vi "status.vi"(8 "error in (no error)":errorcluster, 11 "EventDaemon in":refnum<class "MemoryManager.lvclass">) -> (0 "error out":errorcluster, 2 "status":T1, 3 "EventDaemon out":refnum<class "MemoryManager.lvclass">)   [LabVIEW 2024, in "MemoryManager.lvclass"]
doc: "Get current status and send via notifier."
uses:
  MemoryManager.lvclass
  status--cluster.ctl
  states--enum.ctl
  MemoryManager.lvclass/MemoryManager.ctl
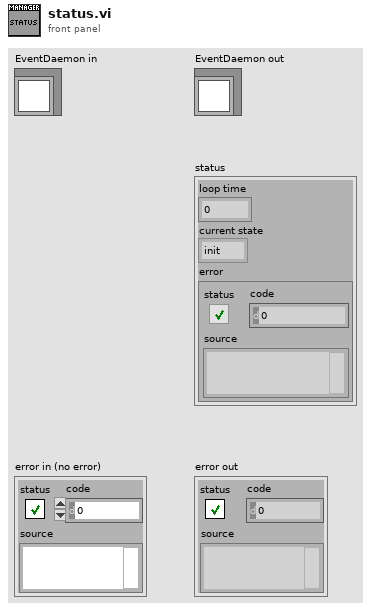
[diagram p1: front panel]
types:
  T1 = typedef "MemoryManager.lvclass/status--cluster.ctl" = cluster{"loop time":u32, "current state":T2, "error":errorcluster}
  T2 = typedef "MemoryManager.lvclass/states--enum.ctl" = enum16{"init", "default", "error handler", "exit"}
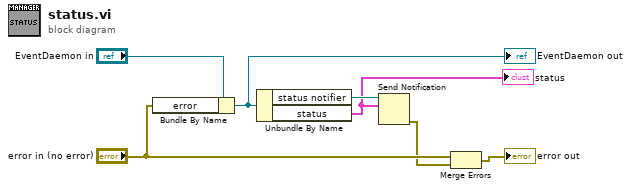
[diagram p0: block diagram]
diagram:
  n1 = Bundle By Name(cluster="EventDaemon in", "error"="error in (no error)") -> (w4:refnum<class "MemoryManager.lvclass">)
  "EventDaemon out" <- w4
  n2 = Unbundle By Name(w4) -> ("status notifier"=w7:refnum<notifier>, "status"=w6:T1)
  "status" <- w6
  n3 = Send Notification(notification=w6, notifier=w7) -> (error out=w1:errorcluster)  [unwired: 1 in, 1 out]
  n4 = Merge Errors("error in (no error)", w1) -> (→"error out":errorcluster)
